vi "Scale All Parameter Constraints.vi"(7 "Fit Model":T1 caption="Model", 8 "Error In":errorcluster, 9 "Normalization Factor":dbl, 11 "parameter bounds in (w tau)":T2) -> (0 "Error Out":errorcluster, 3 "parameter bounds out (w sigma)":T2)   [LabVIEW 2021, in "Fits.lvlib"]
doc: "The VI expects that bounfs for all parameters of the model are provided.\n\nThis VI assumes that the <B>Fit Parameter Constraints</B> involve tau, and returns values which involve sigma = sqrt(tau).\n\nRescales the constraints according to the Y normalization factor."
uses:
  Fits.lvlib
  Decay Convolution/Decay Model.ctl
  <vilib>/Utility/error.llb/Error Cluster From Error Code.vi
  <vilib>/ErrorRing/Error Ring.xnode
panel:
  # "returns sigma = sqrt(abs(tau))"
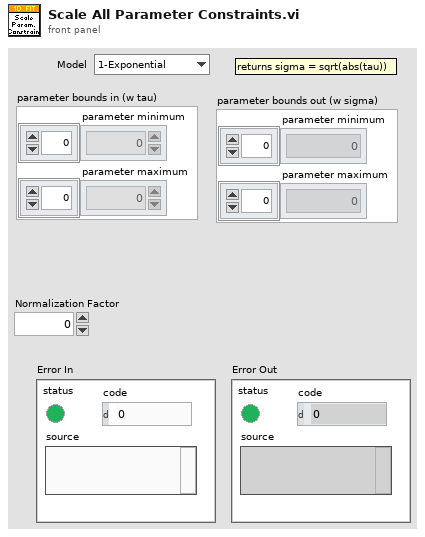
[diagram p1: front panel]
types:
  T1 = typedef "Fits.lvlib/Decay Model.ctl" = enum16{"1-Exponential", "2-Exponentials"}
  T2 = cluster{"parameter minimum":dbl[], "parameter maximum":dbl[]}
  T3 = typedef "Fits.lvlib/Decay Fit Parameters In List.ctl" = enum16{"Offset", "Baseline", "A_1", "tau_1", "A_2", "tau_2"}
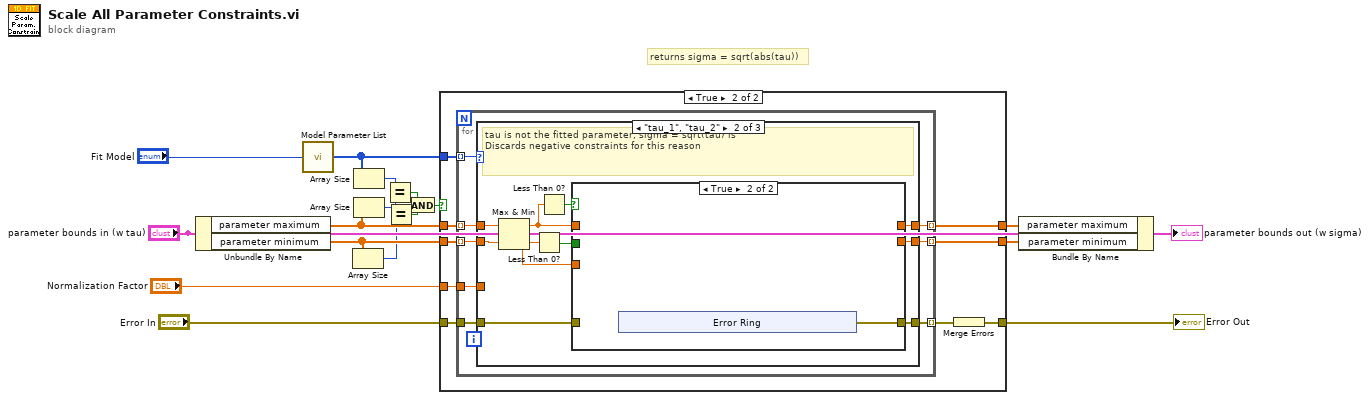
[diagram p0: block diagram]
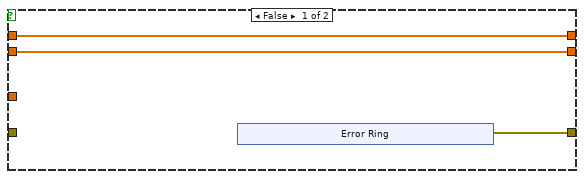
[diagram p2: hidden frame]
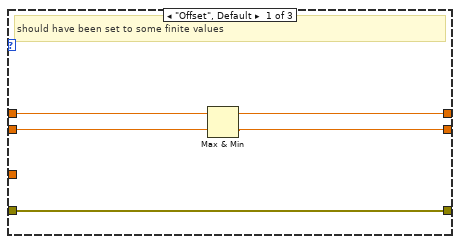
[diagram p3: hidden frame]
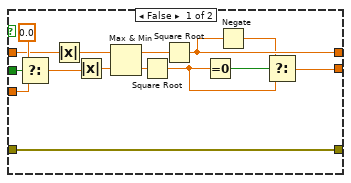
[diagram p4: hidden frame]
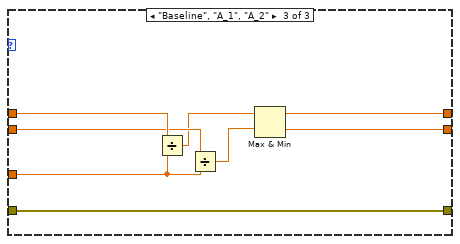
[diagram p5: hidden frame]
diagram:
  # "returns sigma = sqrt(abs(tau))"
  n1 = Unbundle By Name("parameter bounds in (w tau)") -> ("parameter maximum"=w10:dbl[], "parameter minimum"=w9:dbl[])
  n2 = call "Model Parameter List.vi"("Fit Model"="Fit Model") -> ("Model Parameter List"=w12:T3[])
  n3 = Array Size(array=w9) -> (size(s)=w6:i32)
  n4 = Array Size(array=w12) -> (size(s)=w8:i32)
  n5 = Array Size(array=w10) -> (size(s)=w7:i32)
  n6 = Equal?(x=w8, y=w7) -> (x = y?=w5:bool)
  n7 = Equal?(x=w7, y=w6) -> (x = y?=w4:bool)
  n8 = And(x=w5, y=w4) -> (x .and. y?=w3:bool)
  n9 = case shown="True" w3 {
    tunnel: "Normalization Factor" -> [_ w33]
    tunnel: [w20 w32] -> w16
    tunnel: [w19 w31] -> w15
    tunnel: w12 -> [_ w30]
    tunnel: w10 -> [w20 w29]
    tunnel: w9 -> [w19 w28]
    tunnel: "Error In" -> [_ w27]
    tunnel: [w18 w25] -> w1
    frame False {
      n10 = xnode "Error Ring"() -> ("error out"=w18:errorcluster)
    }
    frame True {
      n11 = for {
        tunnel: w29 -> [w39] mode=indexing
        tunnel: w30 -> [w41] mode=indexing
        tunnel: w33 -> [w40]
        tunnel: w28 -> [w38] mode=indexing
        tunnel: [w37] -> w32 mode=indexing
        tunnel: [w36] -> w31 mode=indexing
        tunnel: w27 -> [w35]
        tunnel: [w34] -> w26 mode=indexing
        n12 = case shown="\"tau_1\", \"tau_2\"" w41 {
          tunnel: w40 -> [_ _ w82]
          tunnel: w39 -> [w46 w54 w84]
          tunnel: w38 -> [w45 w53 w83]
          tunnel: [w44 w55 w79] -> w37
          tunnel: [w43 w56 w78] -> w36
          tunnel: w35 -> [w42 w47 w77]
          tunnel: [w42 w49 w77] -> w34
          frame "Offset", Default {
            # "should have been set to some finite values"
            n13 = Max & Min(x=w46, y=w45) -> (max(x,y)=w44:dbl, min(x,y)=w43:dbl)
          }
          frame "tau_1", "tau_2" {
            # "tau is not the fitted parameter, sigma = sqrt(tau) is\nDiscards negative constraints for this reason"
            n14 = Max & Min(x=w54, y=w53) -> (max(x,y)=w50:dbl, min(x,y)=w51:dbl)
            n15 = Less Than 0?(x=w51) -> (x < 0?=w52:bool)
            n16 = Less Than 0?(x=w50) -> (x < 0?=w48:bool)
            n17 = case shown="True" w48 {
              tunnel: [w66 _] -> w56
              tunnel: [w64 _] -> w55
              tunnel: w52 -> [w62 _]
              tunnel: w51 -> [w61 _]
              tunnel: w50 -> [w58 _]
              tunnel: [w57 w72] -> w49
              tunnel: w47 -> [w57 _]
              frame False {
                n18 = Select(t=0.0, s=w62, f=w61) -> (s? t:f=w59:dbl)
                n19 = Absolute Value(x=w58) -> (abs(x)=w71:dbl)
                n20 = Absolute Value(x=w59) -> (abs(x)=w70:dbl)
                n21 = Max & Min(x=w71, y=w70) -> (max(x,y)=w69:dbl, min(x,y)=w68:dbl)
                n22 = Square Root(x=w68) -> (sqrt(x)=w65:dbl)
                n23 = Square Root(x=w69) -> (sqrt(x)=w64:dbl)
                n24 = Equal To 0?(x=w65) -> (x = 0?=w67:bool)
                n25 = Negate(x=w64) -> (-x=w63:dbl)
                n26 = Select(t=w63, s=w67, f=w65) -> (s? t:f=w66:dbl)
              }
              frame True {
                n27 = xnode "Error Ring"() -> ("error out"=w72:errorcluster)
              }
            }
          }
          frame "Baseline", "A_1", "A_2" {
            n28 = Divide(x=w84, y=w82) -> (x/y=w81:dbl)
            n29 = Divide(x=w83, y=w82) -> (x/y=w80:dbl)
            n30 = Max & Min(x=w81, y=w80) -> (max(x,y)=w79:dbl, min(x,y)=w78:dbl)
          }
        }
      }
      n31 = Merge Errors(w26) -> (w25:errorcluster)
    }
  }
  "Error Out" <- w1
  n32 = Bundle By Name(cluster="parameter bounds in (w tau)", "parameter maximum"=w16, "parameter minimum"=w15) -> (→"parameter bounds out (w sigma)":T2)
